vi "Program Oscillator.vi"() -> ()   [LabVIEW 2012]
uses:
  Type/_RT Command.ctl
  <vilib>/Utility/config.llb/Read Key (U32).vi
  Configuration/_Global Configuration.vi
  <vilib>/Utility/config.llb/Write Key (Double).vi
  <vilib>/Utility/config.llb/Write Key (String).vi
  <vilib>/Utility/config.llb/Read Key (Double).vi
  <vilib>/Utility/config.llb/Write Key (U32).vi
  <vilib>/Utility/config.llb/NI_LVConfig.lvlib
panel:
  in  "Chip Select":u32(ring) items=["Q1-FREQ", "Q2-FREQ", "MP1-FREQ"]
  out "Register 0,1,6,7":u32=2764113333
  in  "Program":bool
  out "Frequency Tuning Word":u32=1073741824
  out "Register 7":u8=181 format="%.0x"
  out "Register 6":u8=5 format="%.0x"
  out "Register 5":u8 format="%.0x"
  out "Register 4":u8 format="%.0x"
  out "Register 3":u8 format="%.0x"
  out "Register 2":u8=64 format="%.0x"
  out "Register 1":u8=193 format="%.0x"
  out "Register 0":u8=164 format="%.0x"
  in  "Amplitude Scale Factor":dbl=0.6 min=0.0 max=1.9921875 format="%#.8g"
  in  "Frequency Out (MHz)":dbl=1.0 min=0.0 max=1000.0 format="%#.8g"
  in  "Reference Clock Multiplier":dbl=10.0 min=4.0 max=20.0 step=1.0 format="%#.8g"
  in  "Reference Clock (MHz)":dbl=10.0 min=0.0 max=1000.0 format="%#.8g"
  # "Warning: The values below do not necessary represent the current instrument settings."
  # "(160 + the Reference Clock Multipler value)"
  # "(193, the value to select single tone mode, DPD pin for shutdown, no SLEEP mode)"
  # "(the 1st 8 bits of the frequency tuning word)"
  # "(the 2nd 8 bits of the frequency tuning word)"
  # "(the 3rd 8 bits of the frequency tuning word)"
  # "(the last 8 bits of the frequency tuning word)"
  # "(5, the value to bypass the CIC filter)"
  # "(128 * the Amplitude Scale Factor)"
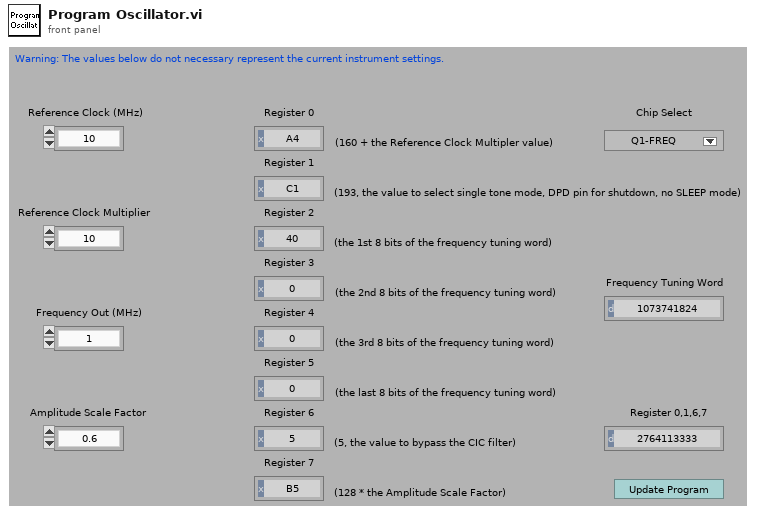
[diagram p1: front panel]
types:
  T1 = typedef "_RT Command.ctl" = enum16{"Start", "Stop", "Runtime Update", "Get Data", "Get Info", "Get Status", "Get Param", "Get Config", "Get Table", "Read ADC", "Set Oscillator", "Update Config", "Update Table", "Set All Pol", "Set Pol and DC", "Set Max Mass", "Toggle RP", "Toggle EL", "Set PIC", "Initialize Turbo", "Send Turbo Comm", "Close Turbo", "P1", "P2", "P3", "Send Serial", "Set LC Out", "Get LC In", "Read VAC", "Test Table", "Toggle Power", "Get Startup", "Set Startup", "Get ADC Table", "Set ADC Table", "Get Brief Status", "Get Detail Status", "Auxiliary Update", "Set CC Logics", "Set CC Input Logics", "Ignore Error"}
  T2 = typedef "NI_LVConfig.lvlib/Config Data RefNum.ctl" = refnum<k1>
  T3 = typedef "_RT Instrument 2.ctl" = cluster{"Table":T4[], "Instrument":string[]}
  T4 = typedef "_RT Configuration 2.ctl" = cluster{"Name":string, "Ch#":u8, "Min":dbl, "Max":dbl, "Def+":dbl, "Def-":dbl, "Offset":dbl, "Slope":dbl, "Type":u8, "Description":string, "SettleT":dbl}
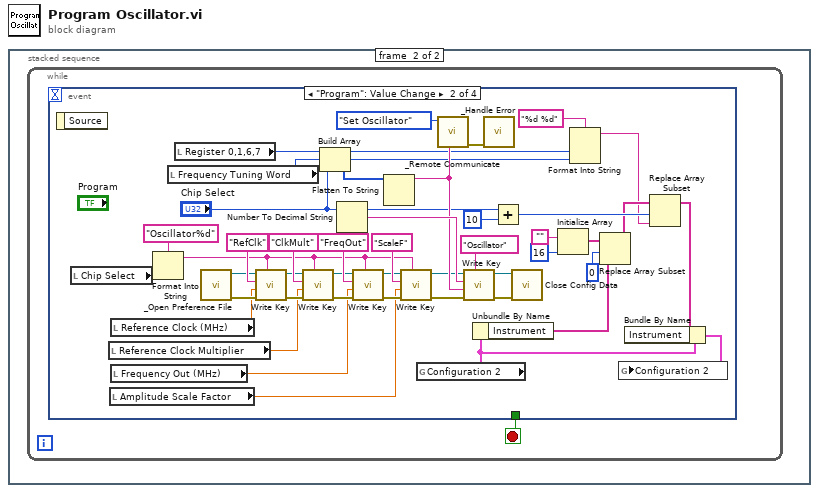
[diagram p0: block diagram]
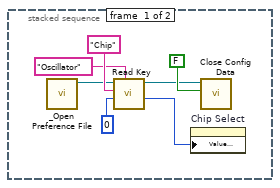
[diagram p2: hidden frame]
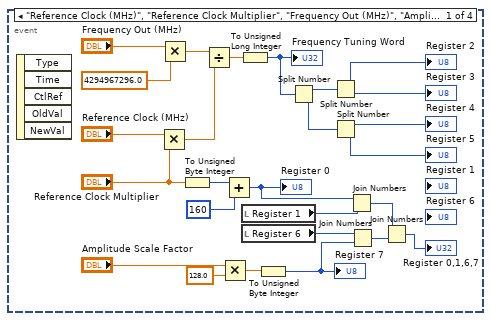
[diagram p3: hidden frame]
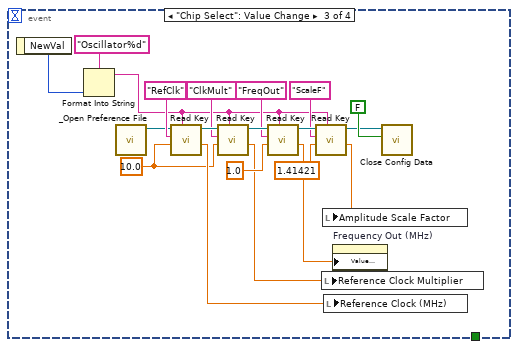
[diagram p4: hidden frame]
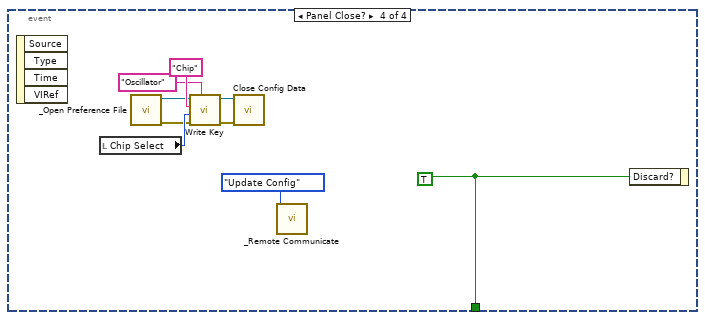
[diagram p5: hidden frame]
diagram:
  n1 = stacked-sequence {
    frame #0 {
      n2 = call "_Open Preference File.vi"() -> ("refnum"=w2:T2)  [unwired: 1 in, 6 out]
      n3 = call-poly <vilib>:"Read Key.vi"("section"="Oscillator", "default value"=u32 0 ("Chip Select"), "key"="Chip" ("section"), "refnum"=w2) -> ("value"=w3:u32, "refnum out"=w5:T2)  [unwired: 1 in, 5 out]
      n4 = property on="Chip Select" class="Ring (strict)"("Value (Signaling)"=w3) -> ()  [unwired: 2 in, 2 out]
      n5 = call <vilib>:"Close Config Data.vi"("write file if changed (T)"=FALSE ("write configuration file? (T)"), "refnum"=w5) -> ()  [unwired: 1 in, 9 out]
    }
    frame #1 {
      n6 = while {
        stop <- w8 stop-if-true
        n7 = event shown="[1] \"Program\": Value Change" {
          selector: _ -> [_ _ _ _]
          dyn-events: _ -> [_ _ _ _]
          timeout: _ -> [_ _ _ _]
          tunnel: [_ _ _ w108] -> w8
          event "Reference Clock (MHz)", "Reference Clock Multiplier", "Frequency Out (MHz)", "Amplitude Scale Factor": Value Change {
            n8 = event-data() -> ()  [unwired: 6 out]
            n9 = Multiply(x="Reference Clock (MHz)", y="Reference Clock Multiplier") -> (x*y=w30:dbl)
            n10 = Multiply(x="Frequency Out (MHz)", y=4294967296.0) -> (x*y=w31:dbl)
            n11 = To Unsigned Byte Integer(number="Reference Clock Multiplier") -> (unsigned 8bit integer=w19:u8)
            n12 = Divide(x=w31, y=w30) -> (x/y=w29:dbl)
            n13 = Multiply(x="Amplitude Scale Factor", y=128.0) -> (x*y=w18:dbl)
            n14 = Add(x=w19, y=u8 160) -> (x+y=w15:u8)
            "Register 0" <- w15
            n15 = To Unsigned Long Integer(number=w29) -> (unsigned 32bit integer=w28:u32)
            "Frequency Tuning Word" <- w28
            n16 = local read "Register 1"() -> (w14:u8)
            n17 = local read "Register 6"() -> (w11:u8)
            n18 = To Unsigned Byte Integer(number=w18) -> (unsigned 8bit integer=w9:u8)
            "Register 7" <- w9
            n19 = Split Number(x=w28) -> (hi(x)=w27:u16, lo(x)=w26:u16)
            n20 = Split Number(x=w27) -> (hi(x)=→"Register 2":u8, lo(x)=→"Register 3":u8)
            n21 = Split Number(x=w26) -> (hi(x)=→"Register 4":u8, lo(x)=→"Register 5":u8)
            n22 = Join Numbers(hi=w15, lo=w14) -> ((hi.lo)=w13:u16)
            n23 = Join Numbers(hi=w11, lo=w9) -> ((hi.lo)=w12:u16)
            n24 = Join Numbers(hi=w13, lo=w12) -> ((hi.lo)=→"Register 0,1,6,7":u32)
          }
          event "Program": Value Change {
            n25 = event-data() -> ()  [unwired: 2 out]
            n26 = local read "Chip Select"() -> (w52:u32)
            n27 = local read "Reference Clock Multiplier"() -> (w58:dbl)
            n28 = local read "Amplitude Scale Factor"() -> (w56:dbl)
            n29 = local read "Reference Clock (MHz)"() -> (w59:dbl)
            n30 = local read "Frequency Out (MHz)"() -> (w57:dbl)
            n31 = Format Into String(format string="Oscillator%d", w52) -> (resulting string=w51:string)  [unwired: 2 in, 1 out]
            n32 = local read "Frequency Tuning Word"() -> (w48:u32)
            n33 = local read "Register 0,1,6,7"() -> (w49:u32)
            n34 = call "_Open Preference File.vi"() -> ("error"=w68:errorcluster, "refnum"=w63:T2)  [unwired: 1 in, 5 out]
            n35 = call-poly <vilib>:"Write Key.vi"("section"=w51, "error in (no error)"=w68, "value"=w59, "key"="RefClk" ("section"), "refnum"=w63) -> ("error out"=w69:errorcluster, "refnum out"=w62:T2)  [unwired: 3 in, 2 out]
            n36 = call-poly <vilib>:"Write Key.vi"("section"=w51, "error in (no error)"=w69, "value"=w58, "key"="ClkMult" ("section"), "refnum"=w62) -> ("error out"=w70:errorcluster, "refnum out"=w61:T2)  [unwired: 3 in, 2 out]
            n37 = Build Array(w49, w48, "Chip Select") -> (w79:u32[])
            n38 = Number To Decimal String(number="Chip Select") -> (decimal integer string=w75:string)  [unwired: 1 out]
            n39 = call-poly <vilib>:"Write Key.vi"("section"=w51, "error in (no error)"=w70, "value"=w57, "key"="FreqOut" ("section"), "refnum"=w61) -> ("error out"=w71:errorcluster, "refnum out"=w60:T2)  [unwired: 3 in, 2 out]
            n40 = Flatten To String(anything=w79) -> (data string=w74:string)  [unwired: 1 in, 4 out]
            n41 = call-poly <vilib>:"Write Key.vi"("section"=w51, "error in (no error)"=w71, "value"=w56, "key"="ScaleF" ("section"), "refnum"=w60) -> ("error out"=w54:errorcluster, "refnum out"=w55:T2)  [unwired: 3 in, 2 out]
            n42 = global read "_Global Configuration.vi" "Configuration 2"() -> (w50:T3)
            n43 = call "_Remote Communicate.vi"("String"=w74, "Command"=_RT_Command."Set Oscillator") -> ("error out"=w77:errorcluster)  [unwired: 4 in, 3 out]
            n44 = call-poly <vilib>:"Write Key.vi"("section"="Oscillator", "error in (no error)"=w54, "value"=w74, "key"=w75, "refnum"=w55) -> ("error out"=w72:errorcluster, "refnum out"=w73:T2)  [unwired: 1 in, 4 out]
            n45 = Unbundle By Name(w50) -> ("Instrument"=w39:string[])
            n46 = call "_Handle Error.vi"("error in (no error)"=w77) -> ()  [unwired: 2 in, 5 out]
            n47 = Add(x="Chip Select", y=u32 10) -> (x+y=w42:u32)
            n48 = call <vilib>:"Close Config Data.vi"("error in (no error)"=w72, "refnum"=w73) -> ()  [unwired: 1 in, 9 out]
            n49 = Initialize Array("", 16 ("dimension size")) -> (w41:string[])
            n50 = Format Into String(format string="%d %d", w49, w48) -> (resulting string=w37:string)  [unwired: 2 in, 1 out]
            n51 = Replace Array Subset(array=w41, new element=w39, index=0) -> (w38:string[])
            n52 = Replace Array Subset(array=w38, new element=w37, index=w42) -> (w36:string[])
            n53 = Bundle By Name(cluster=w50, "Instrument"=w36) -> (w35:T3)
            n54 = global write "_Global Configuration.vi" "Configuration 2"(w35) -> ()
          }
          event "Chip Select": Value Change {
            w80 = 10.0 ("Value (Signaling)")
            n55 = event-data() -> ("NewVal"=w84:u32)  [unwired: 1 out]
            n56 = Format Into String(format string="Oscillator%d", w84) -> (resulting string=w82:string)  [unwired: 2 in, 1 out]
            n57 = call "_Open Preference File.vi"() -> ("refnum"=w98:T2)  [unwired: 1 in, 6 out]
            n58 = call-poly <vilib>:"Read Key.vi"("section"=w82, "default value"=w80, "key"="RefClk" ("section"), "refnum"=w98) -> ("value"=w87:dbl, "refnum out"=w97:T2)  [unwired: 1 in, 5 out]
            n59 = call-poly <vilib>:"Read Key.vi"("section"=w82, "default value"=w80, "key"="ClkMult" ("section"), "refnum"=w97) -> ("value"=w88:dbl, "refnum out"=w96:T2)  [unwired: 1 in, 5 out]
            n60 = call-poly <vilib>:"Read Key.vi"("section"=w82, "default value"=1.0 ("Value (Signaling)"), "key"="FreqOut" ("section"), "refnum"=w96) -> ("value"=w89:dbl, "refnum out"=w95:T2)  [unwired: 1 in, 5 out]
            n61 = call-poly <vilib>:"Read Key.vi"("section"=w82, "default value"=1.41421 ("Value (Signaling)"), "key"="ScaleF" ("section"), "refnum"=w95) -> ("value"=w85:dbl, "refnum out"=w81:T2)  [unwired: 1 in, 5 out]
            n62 = local write "Reference Clock Multiplier"(w88) -> ()
            n63 = local write "Amplitude Scale Factor"(w85) -> ()
            n64 = local write "Reference Clock (MHz)"(w87) -> ()
            n65 = property on="Frequency Out (MHz)" class="DigNum (strict)"("Value (Signaling)"=w89) -> ()  [unwired: 2 in, 2 out]
            n66 = call <vilib>:"Close Config Data.vi"("write file if changed (T)"=FALSE ("write configuration file? (T)"), "refnum"=w81) -> ()  [unwired: 1 in, 9 out]
          }
          event Panel Close? {
            w108 = TRUE
            n67 = event-data() -> ()  [unwired: 5 out]
            n68 = local read "Chip Select"() -> (w104:u32)
            n69 = call "_Open Preference File.vi"() -> ("error"=w101:errorcluster, "refnum"=w102:T2)  [unwired: 1 in, 5 out]
            n70 = call-poly <vilib>:"Write Key.vi"("section"="Oscillator", "error in (no error)"=w101, "value"=w104, "key"="Chip" ("section"), "refnum"=w102) -> ("error out"=w106:errorcluster, "refnum out"=w105:T2)  [unwired: 5 out]
            n71 = call <vilib>:"Close Config Data.vi"("error in (no error)"=w106, "refnum"=w105) -> ()  [unwired: 1 in, 9 out]
            n72 = call "_Remote Communicate.vi"("Command"=_RT_Command."Update Config") -> ()  [unwired: 5 in, 4 out]
            n73 = event-data("Discard?"=w108) -> ()  [unwired: 1 in, 1 out]
          }
        }
      }
    }
  }
